vi "binarize.vi"(8 "error in":errorcluster caption="entrée d'erreur", 9 "X":string[][](array[string]), 10 "Type X":T1(ring), 11 "binarize":cluster{"threshold":dbl, "copy":bool}={"threshold"=0.0, "copy"=TRUE}) -> (0 "error out":errorcluster caption="sortie d'erreur", 3 "Data":T2)   [LabVIEW 2020]
doc: "Boolean thresholding of array-like or scipy.sparse matrix\n\n\nParameters :\n\n- X : {array-like, sparse matrix}, shape [n_samples, n_features]\nThe data to binarize, element by element. scipy.sparse matrices should be in CSR or CSC format to avoid an un-necessary copy.\n\n- threshold : float (0.0 by default)\nFeature values below or equal to this are replaced by 0, above it by 1. Threshold may not be less than 0 for operations on sparse matrices.\n\n- copy : boolean, optional, default True\nset to False to perform inplace binarization and avoid a copy (if the input is already a numpy array or a scipy.sparse CSR / CSC matrix and if axis is 1)."
uses:
  binarize.lvclass
panel:
  out "binarize.lvclass":refnum<class "binarize.lvclass">
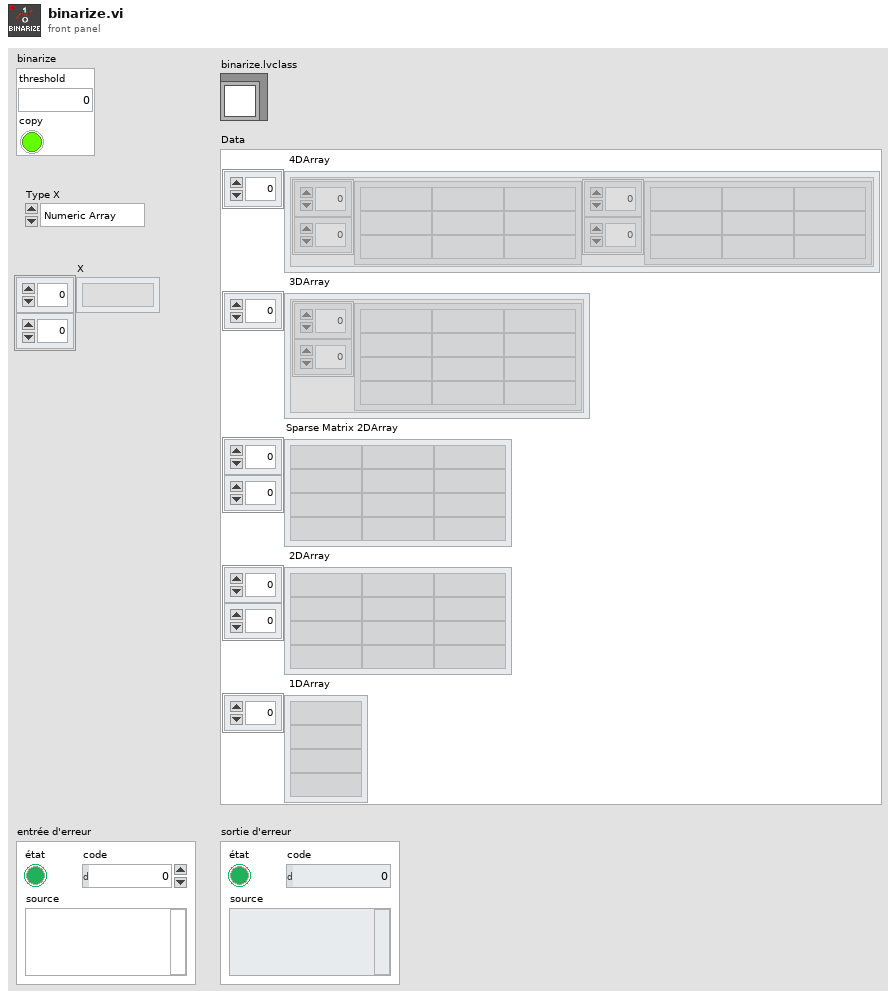
[diagram p1: front panel]
types:
  T1 = enum16{"Numeric Array", "String Array", "Sparse"}
  T2 = cluster{" 4DArray":cluster{"1":string[][], "2":string[][]}[], " 3DArray":cluster{"Tableau":string[][]}[], "Sparse Matrix 2DArray":string[][], " 2DArray":string[][], " 1DArray":string[]}
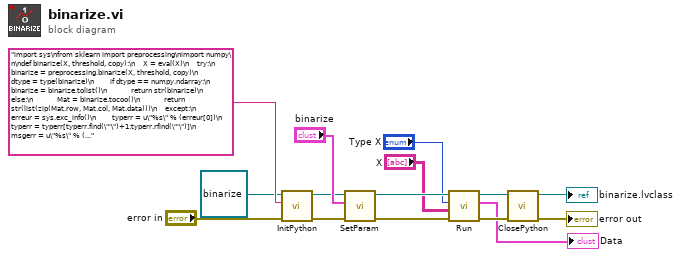
[diagram p0: block diagram]
diagram:
  n1 = call-dynamic "InitPython.vi"("error in (no error)"="error in", "Python Instruction"="import sys\nfrom sklearn import preprocessing\nimport numpy\n\ndef binarize(X, threshold, copy):\n    X = eval(X)\n    try:\n        binarize = preprocessing.binarize(X, threshold, copy)\n        dtype = type(binarize)\n        if dtype == numpy.ndarray:\n            binarize = binarize.tolist()\n            return str(binarize)\n        else:\n            Mat = binarize.tocoo()\n            return str(list(zip(Mat.row, Mat.col, Mat.data)))\n    except:\n        erreur = sys.exc_info()\n        typerr = u\"%s\" % (erreur[0])\n        typerr = typerr[typerr.find(\"'\")+1:typerr.rfind(\"'\")]\n        msgerr = u\"%s\" % (erreur[1])\n        message = str('/!\\\\ {0} : {1}'. format(typerr,msgerr))\n        return message", "Scikit-learn en entrée"=refnum<class "binarize.lvclass"> refnum ("binarize.lvclass")) -> ("error out"=w10:errorcluster, "Scikit-learn en sortie"=w8:refnum<class "binarize.lvclass">)  [unwired: 7 in]
  n2 = call-dynamic "SetParam.vi"("error in (no error)"=w10, "binarize"="binarize", "binarize.lvclass"=w8) -> ("error out"=w5:errorcluster, "binarize.lvclass"=w7:refnum<class "binarize.lvclass">)  [unwired: 7 in]
  n3 = call-dynamic "Run.vi"("error in (no error)"=w5, "X"="X", "Type X"="Type X", "binarize.lvclass"=w7) -> ("error out"=w3:errorcluster, "Data"=→"Data":T2, "binarize.lvclass"=w4:refnum<class "binarize.lvclass">)  [unwired: 5 in]
  n4 = call-dynamic "ClosePython.vi"("error in (no error)"=w3, "Scikit-learn en entrée"=w4) -> ("error out"=→"error out":errorcluster, "Scikit-learn en sortie"=→"binarize.lvclass":refnum<class "binarize.lvclass">)  [unwired: 8 in]
